vi "Handle Variable Header.vi"(8 "error in (no error)":errorcluster, 10 "Incoming Packets":u8[](array[numeric]) format="%08b", 11 "ControlPacket in":refnum<class "ControlPacket.lvclass">) -> (0 "error out":errorcluster, 1 "Variable Header Complete?":bool=TRUE, 2 "Remaining Packets":u8[](array[numeric]) format="%08b", 3 "ControlPacket out":refnum<class "ControlPacket.lvclass">)   [LabVIEW 2013, in "MQTT_Control_Packets.lvlib" / "ControlPacket.lvclass"]
uses:
  ControlPacket.lvclass
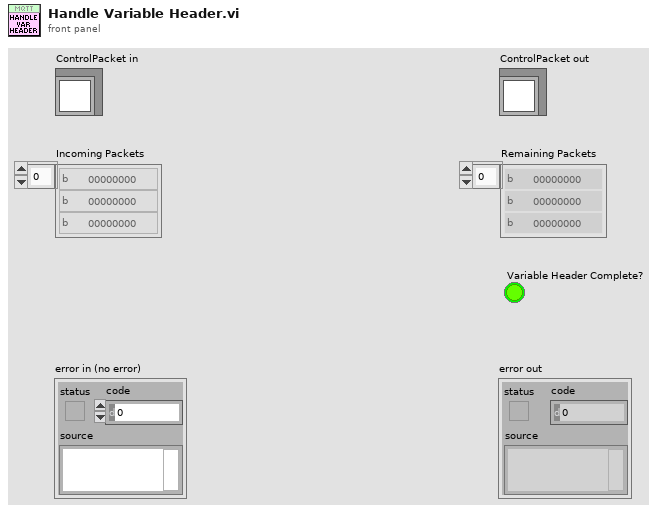
[diagram p1: front panel]
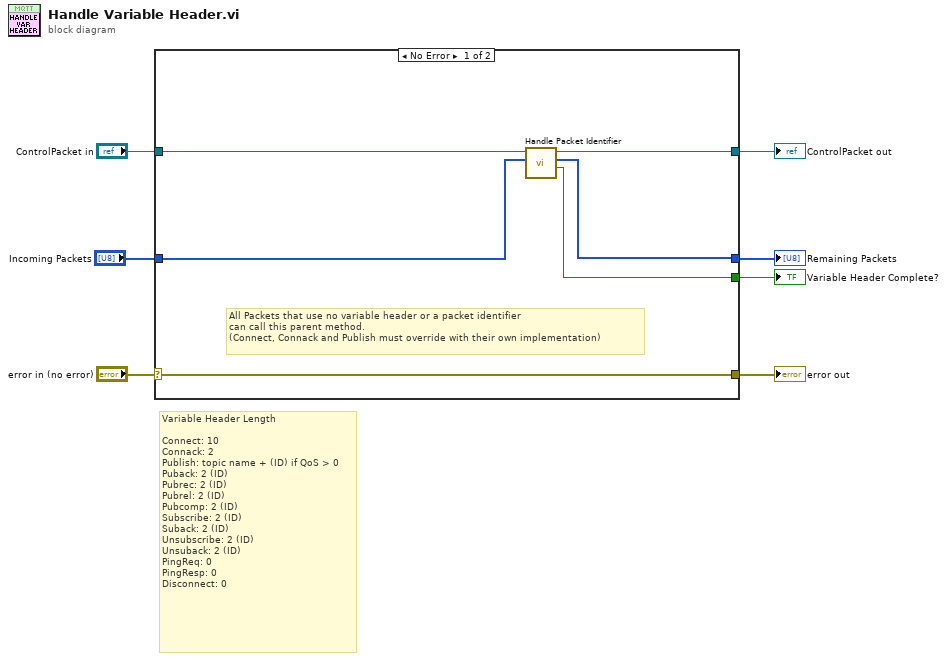
[diagram p0: block diagram]
diagram:
  # "Variable Header Length\n\nConnect: 10\nConnack: 2\nPublish: topic name + (ID) if QoS > 0\nPuback: 2 (ID)\nPubrec: 2 (ID)\nPubrel: 2 (ID)\nPubcomp: 2 (ID)\nSubscribe: 2 (ID)\nSuback: 2 (ID)\nUnsubscribe: 2 (ID)\nUnsuback: 2 (ID)\nPingReq: 0\nPingResp: 0\nDisconnect: 0"
  n1 = case shown="No Error" "error in (no error)" {
    selector: "error in (no error)" -> [w13 w16]
    tunnel: [w13 w16] -> w6
    tunnel: [w12 w15] -> w4
    tunnel: "ControlPacket in" -> [w8 w15]
    tunnel: "Incoming Packets" -> [w11 w14]
    tunnel: [w10 w14] -> w2
    tunnel: [w9 _] -> w1
    frame No Error {
      # "All Packets that use no variable header or a packet identifier\ncan call this parent method.\n(Connect, Connack and Publish must override with their own implementation)"
      n2 = call "Handle Packet Identifier.vi"("Incoming Packets"=w11, "ControlPacket in"=w8) -> ("Identifier Complete?"=w9:bool, "Remaining Packets"=w10:u8[], "ControlPacket out"=w12:refnum<class "ControlPacket.lvclass">)  [unwired: 6 in, 1 out]
    }
    frame Error {
    }
  }
  "error out" <- w6
  "ControlPacket out" <- w4
  "Remaining Packets" <- w2
  "Variable Header Complete?" <- w1
